vi "Data_Record_Example.vi"() -> ()   [LabVIEW 2021]
uses:
  <vilib>/Galil/resources/gclib/gclib.lvlib
panel:
  out "TTA":dbl
  out "TIME":u16
  out "TPA":i32
  out "RPA":i32
  in  "IP Address":string="192.168.1.77 --subscribe DR "
  out "error out":errorcluster
  in  "stop":bool
  # "This example is built for the DMC-4000. If you have a different controller, check your controller's User Manual to ensure that the Data Record mapping is correct before running this program."
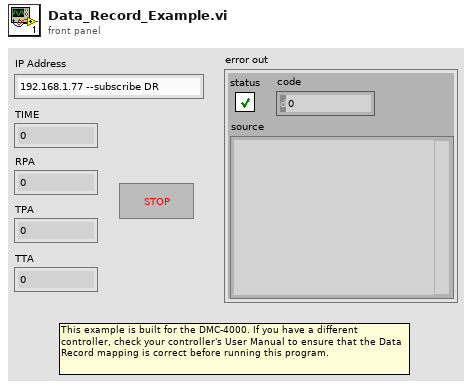
[diagram p1: front panel]
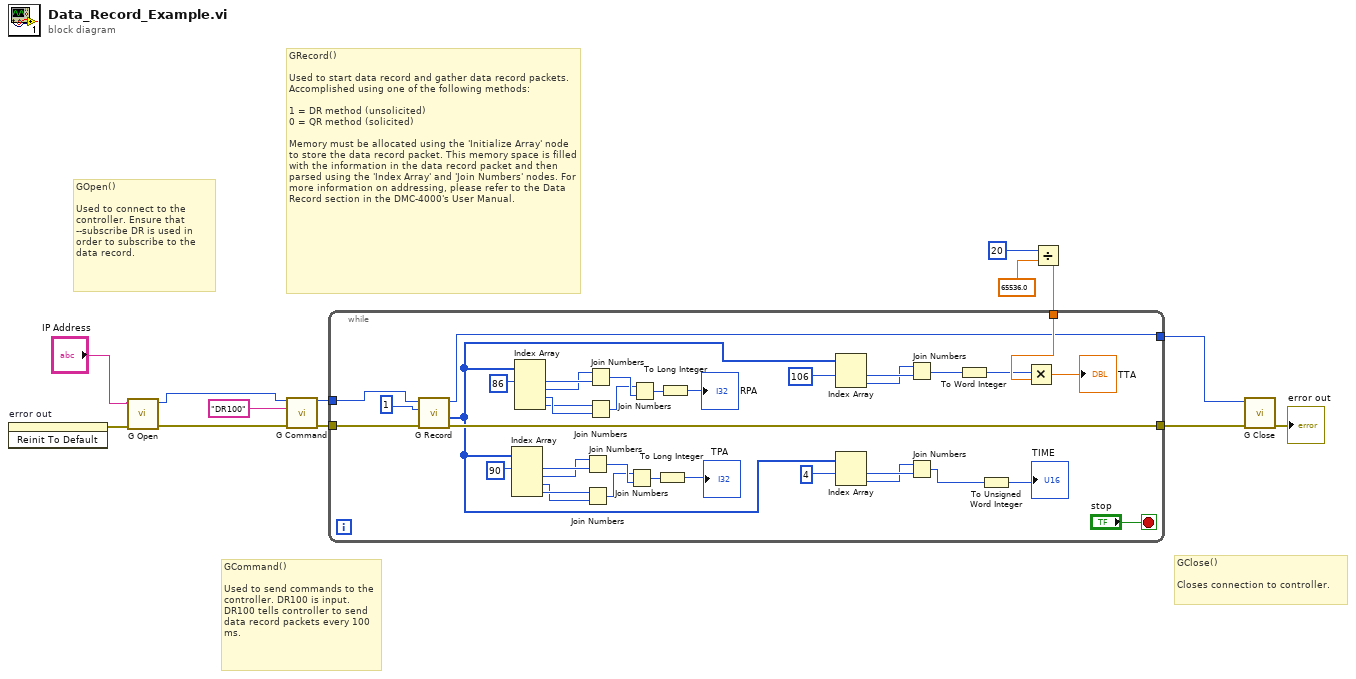
[diagram p0: block diagram]
diagram:
  # "GRecord()\n\nUsed to start data record and gather data record packets. Accomplished using one of the following methods:\n\n1 = DR method (unsolicited)\n0 = QR method (solicited)\n\nMemory must be allocated using the 'Initialize Array' node to store the data record packet. This memory space is filled with the information in the data record packet and then parsed using the 'Index Array' and 'Join Numbers' nodes. For more information on addressing, please refer to the Data Record section in the DMC-4000's User Manual."
  # "GClose()\n\nCloses connection to controller."
  # "GCommand()\n\nUsed to send commands to the controller. DR100 is input. DR100 tells controller to send data record packets every 100 ms."
  # "GOpen()\n\nUsed to connect to the controller. Ensure that \n--subscribe DR is used in order to subscribe to the data record."
  n1 = invoke on="error out" class="Clust (strict)" method="Reinit To Default"() -> (error out=w7:errorcluster)  [unwired: 3 in, 2 out]
  n2 = call <vilib>:"G Open.vi"("error in (no error)"=w7, "address"="IP Address") -> ("error out"=w4:errorcluster, "g out"=w6:u64)  [unwired: 7 in]
  n3 = call <vilib>:"G Command.vi"("g"=w6, "command"="DR100", "error in (no error)"=w4) -> ("g out"=w9:u64, "error out"=w3:errorcluster)  [unwired: 10 in, 1 out]
  n4 = Divide(x=20, y=65536.0) -> (x/y=w10:dbl)
  n5 = while {
    tunnel: [w19] -> w1
    tunnel: w9 -> [w21]
    tunnel: w3 -> [w20]
    tunnel: [w18] -> w2
    tunnel: w10 -> [w23]
    stop <- "stop" stop-if-true
    n6 = call <vilib>:"G Record.vi"("error in (no error)"=w20, "method"=1, "g"=w21) -> ("error out"=w19:errorcluster, "record out"=w17:u8[], "g out"=w18:u64)  [unwired: 6 in]
    n7 = Index Array "Index Array"(array=w17, index #1=90 ("index")) -> (element #1=w43:u8, element #2=w42:u8, element #3=w37:u8, element #4=w40:u8)  [unwired: 3 in]
    n8 = Index Array "Index Array"(array=w17, index #1=86 ("index")) -> (element #1=w49:u8, element #2=w48:u8, element #3=w46:u8, element #4=w45:u8)  [unwired: 3 in]
    n9 = Join Numbers(hi=w42, lo=w43) -> ((hi.lo)=w34:u16)
    n10 = Join Numbers(hi=w40, lo=w37) -> ((hi.lo)=w33:u16)
    n11 = Join Numbers(hi=w48, lo=w49) -> ((hi.lo)=w36:u16)
    n12 = Join Numbers(hi=w45, lo=w46) -> ((hi.lo)=w35:u16)
    n13 = Join Numbers(hi=w33, lo=w34) -> ((hi.lo)=w39:u32)
    n14 = Join Numbers(hi=w35, lo=w36) -> ((hi.lo)=w44:u32)
    n15 = To Long Integer(number=w39) -> (32bit integer=→"TPA":i32)
    n16 = To Long Integer(number=w44) -> (32bit integer=→"RPA":i32)
    n17 = Index Array "Index Array"(array=w17, index #1=106 ("index")) -> (element #1=w32:u8, element #2=w31:u8)  [unwired: 1 in]
    n18 = Index Array "Index Array"(array=w17, index #1=4 ("index")) -> (element #1=w29:u8, element #2=w28:u8)  [unwired: 1 in]
    n19 = Join Numbers(hi=w31, lo=w32) -> ((hi.lo)=w24:u16)
    n20 = Join Numbers(hi=w28, lo=w29) -> ((hi.lo)=w26:u16)
    n21 = To Word Integer(number=w24) -> (16bit integer=w22:i16)
    n22 = To Unsigned Word Integer(number=w26) -> (unsigned 16bit integer=→"TIME":u16)
    n23 = Multiply(x=w22, y=w23) -> (x*y=→"TTA":dbl)
  }
  n24 = call <vilib>:"G Close.vi"("error in (no error)"=w1, "g"=w2) -> ("error out"=→"error out":errorcluster)  [unwired: 9 in]
